vi "ShowUsers.vi"(4 "Sequence Context":T1) -> (0 "error out":errorcluster)   [LabVIEW 2025]
uses:
  <vilib>/addons/TestStand/_TSLegacy.llb/LabVIEW Test - Sequence Context.ctl
panel:
  in  "TS.User":refnum<k7>
  out "Number of Users":i32
  out "Login User Names":string[](array[string])
  in  "?":bool
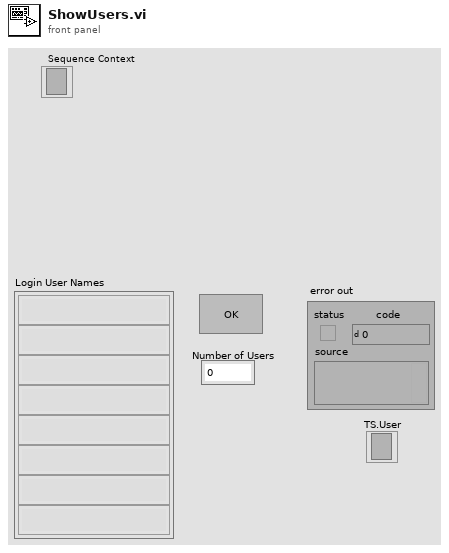
[diagram p1: front panel]
types:
  T1 = typedef "LabVIEW Test - Sequence Context.ctl" = refnum<k7>
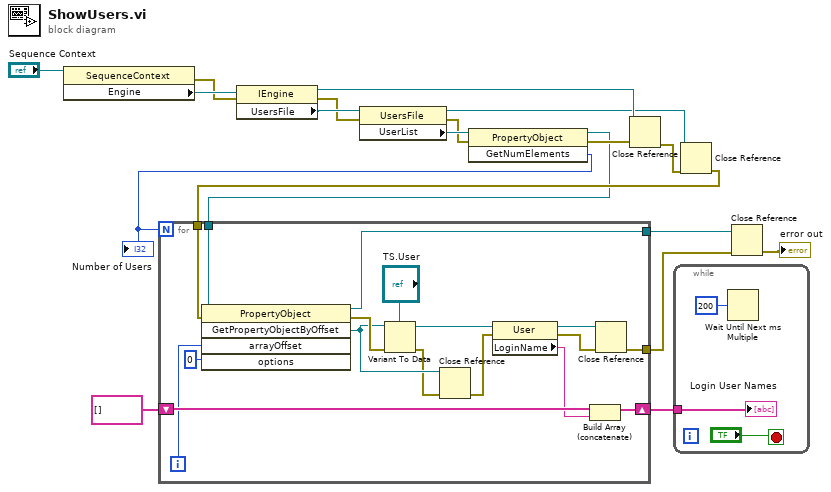
[diagram p0: block diagram]
diagram:
  n1 = property class="SequenceContext"(reference="Sequence Context") -> (error out=w13:errorcluster, "Engine"=w14:refnum<k7>)  [unwired: 1 in, 1 out]
  n2 = property class="IEngine"(reference=w14, error in=w13) -> (reference out=w8:refnum<k7>, error out=w11:errorcluster, "UsersFile"=w12:refnum<k7>)
  n3 = property class="UsersFile"(reference=w12, error in=w11) -> (reference out=w7:refnum<k7>, error out=w9:errorcluster, "UserList"=w10:refnum<k7>)
  n4 = invoke class="PropertyObject" method="GetNumElements"(reference=w10, error in=w9) -> (reference out=w3:refnum<k7>, error out=w6:errorcluster, "GetNumElements"=w5:i32)  [unwired: 1 in]
  "Number of Users" <- w5
  n5 = Close Reference(reference=w8, error in (no error)=w6) -> (error out=w16:errorcluster)
  n6 = Close Reference(reference=w7, error in (no error)=w16) -> (error out=w4:errorcluster)
  n7 = for {
    N: w5 -> [_]
    shift-right: [w36] -> w18
    shift-left: string[] [] -> [w35]
    tunnel: [w34] -> w2
    tunnel: w4 -> [w32]
    tunnel: w3 -> [w33]
    tunnel: [w20] -> w1
    i -> [w31]
    n8 = invoke class="PropertyObject" method="GetPropertyObjectByOffset"(reference=w33, error in=w32, "arrayOffset"=w31, "options"=0) -> (reference out=w20:refnum<k7>, error out=w29:errorcluster, "GetPropertyObjectByOffset"=w26:refnum<k7>)  [unwired: 1 in, 2 out]
    n9 = Variant To Data(error in=w29, type="TS.User", Variant=w26) -> (data=w27:refnum<k7>, error out=w25:errorcluster)
    n10 = Close Reference(reference=w26, error in (no error)=w25) -> (error out=w24:errorcluster)
    n11 = property class="User"(reference=w27, error in=w24) -> (reference out=w23:refnum<k7>, error out=w22:errorcluster, "LoginName"=w21:string)
    n12 = Build Array (concatenate)(w35, w21) -> (w36:string[])
    n13 = Close Reference(reference=w23, error in (no error)=w22) -> (error out=w34:errorcluster)
  }
  n14 = while {
    tunnel: w18 -> [w39]
    stop <- "?" stop-if-true
    n15 = Wait Until Next ms Multiple(millisecond multiple=u32 200) -> ()  [unwired: 1 out]
    "Login User Names" <- w39
  }
  n16 = Close Reference(reference=w1, error in (no error)=w2) -> (error out=→"error out":errorcluster)
